vi "Set_take_data.vi"   [LabVIEW 2010]
uses:
  Globals/Dynamic_call_global.ph.vi
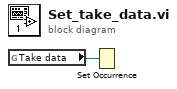
[diagram p0: block diagram]
diagram:
  n1 = global read "Dynamic_call_global.ph.vi" "Take data"() -> (w1:refnum<k4>)
  n2 = Set Occurrence(w1) -> ()
